vi "DAQ Tags.vi"(11 "Tasks":T1[](array[typedef])) -> (3 "DAQ Tags Array":string[](array[string]))   [LabVIEW 2018]
uses:
  Acquisition/Task Cluster.ctl
  <resource>/objmgr/daqmx.rc
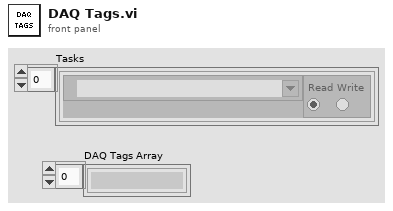
[diagram p1: front panel]
types:
  T1 = typedef "Task Cluster.ctl" = cluster{"DAQmx Task":refnum<k21>, "Read-Write Radio":enum32{"Read", "Write"}}
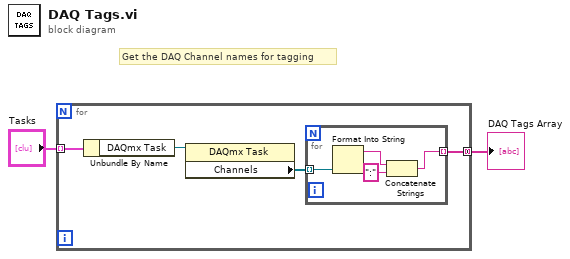
[diagram p0: block diagram]
diagram:
  # "Get the DAQ Channel names for tagging"
  n1 = for {
    tunnel: "Tasks" -> [w5] mode=indexing
    tunnel: [w3] -> w1 mode=concatenating
    n2 = Unbundle By Name(w5) -> ("DAQmx Task"=w6:refnum<k21>)
    n3 = property class="DAQmx Task"(reference=w6) -> ("Channels"=w4:refnum<k21>[])  [unwired: 1 in, 2 out]
    n4 = for {
      tunnel: w4 -> [w10] mode=indexing
      tunnel: [w7] -> w3 mode=indexing
      n5 = Format Into String(w10) -> (resulting string=w9:string)  [unwired: 3 in, 1 out]
      n6 = Concatenate Strings(w9, ":" ("string")) -> (w7:string)
    }
  }
  "DAQ Tags Array" <- w1
